vi "epoch to cluster.vi"() -> ()   [LabVIEW 2024]
uses:
  <vilib>/addons/_JKI.lib/REST Client/classes/REST Client/REST Client.lvclass
panel:
  out "value":T1
  in  "Cluster":T2
  out "Response body":string
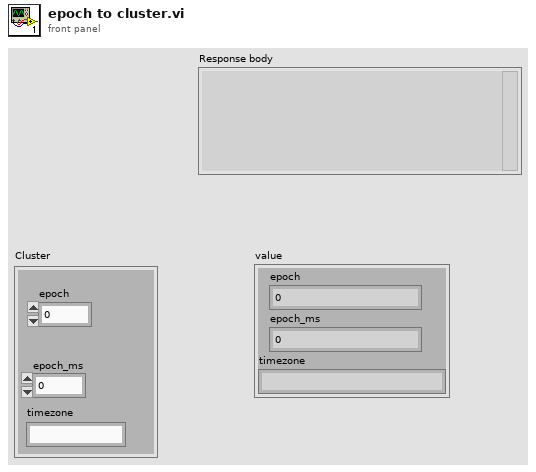
[diagram p1: front panel]
types:
  T1 = cluster{"epoch":dbl, "epoch_ms":dbl, "timezone":string}
  T2 = cluster{"epoch":dbl, "epoch_ms\n":u64, "timezone":string}
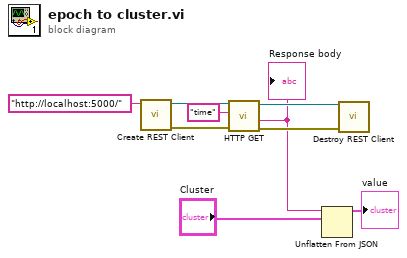
[diagram p0: block diagram]
diagram:
  n1 = call <vilib>:"Create REST Client.vi"("Base URL"="http://localhost:5000/") -> ("error out"=w8:errorcluster, "REST Client out"=w9:refnum<class "REST Client.lvclass">)  [unwired: 9 in]
  n2 = call-dynamic "HTTP GET.vi"("error in (no error)"=w8, "Path"="time", "REST Client in"=w9) -> ("error out"=w6:errorcluster, "Response body"=w3:string, "REST Client out"=w7:refnum<class "REST Client.lvclass">)  [unwired: 3 in, 3 out]
  "Response body" <- w3
  n3 = Unflatten From JSON(JSON string=w3, type and defaults="Cluster") -> (value=→"value":T2)  [unwired: 5 in, 1 out]
  n4 = call-dynamic "Destroy REST Client.vi"("error in (no error)"=w6, "REST Client in"=w7) -> ()  [unwired: 9 in, 1 out]
